vi "Configure Signal.vi"   [LabVIEW 2018]
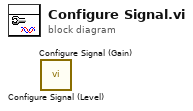
[diagram p0: block diagram]
diagram:
  n1 = call "Configure Signal (Level).vi"() -> ()  [unwired: 9 in, 7 out]
  n2 = call "Configure Signal (Gain).vi"() -> ()  [unwired: 9 in, 7 out]
